vi "GetInstrumentAddr.vi"(1 "String":string) -> (0 "VISA session":refnum<visa-resource-name>, 2 "Instruments":T1(array[cluster]))   [LabVIEW 2013]
uses:
  SourceCode/GlobalValue.vi
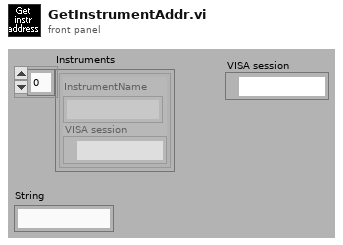
[diagram p1: front panel]
types:
  T1 = cluster{"InstrumentName":string, "VISA session":refnum<visa-resource-name>}[]
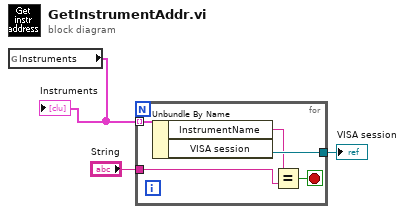
[diagram p0: block diagram]
diagram:
  n1 = global read "GlobalValue.vi" "Instruments"() -> (w1:T1)
  "Instruments" <- w1
  n2 = for {
    tunnel: w1 -> [w8] mode=indexing
    tunnel: [w7] -> w3
    tunnel: "String" -> [w5]
    stop <- w4 stop-if-true
    n3 = Unbundle By Name(w8) -> ("InstrumentName"=w6:string, "VISA session"=w7:refnum<visa-resource-name>)
    n4 = Equal?(x=w6, y=w5) -> (x = y?=w4:bool)
  }
  "VISA session" <- w3
